vi "Init Objects by Type.vi"(8 "error in (no error)":errorcluster, 11 "Application Controller in":refnum<class "Application Controller.lvclass">) -> (0 "error out":errorcluster, 3 "Application Controller out":refnum<class "Application Controller.lvclass">)   [LabVIEW 2016, in "Application Controller.lvclass"]
uses:
  Application Controller.lvclass
  Sequence Elements/Sweep Sequence/Sweep.lvclass
  Sequence Elements/Record/Record.lvclass
  Application Controller.lvclass/Application Controller.ctl
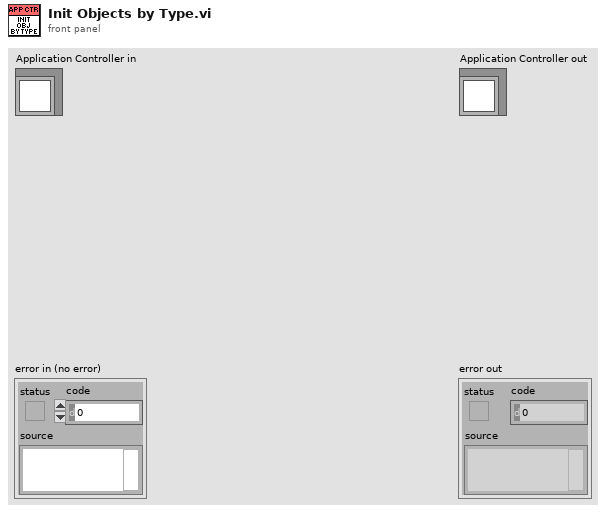
[diagram p1: front panel]
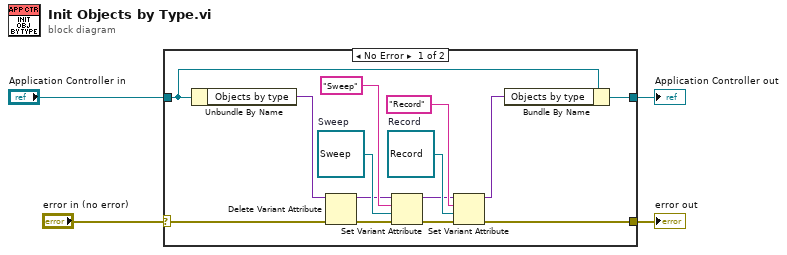
[diagram p0: block diagram]
diagram:
  n1 = case shown="No Error" "error in (no error)" {
    selector: "error in (no error)" -> [w6 w20]
    tunnel: [w5 w20] -> w3
    tunnel: [w8 w19] -> w1
    tunnel: "Application Controller in" -> [w18 w19]
    frame No Error {
      w12 = refnum<class "Record.lvclass"> refnum  # Record
      w16 = refnum<class "Sweep.lvclass"> refnum  # Sweep
      n2 = Unbundle By Name(w18) -> ("Objects by type"=w17:variant)
      n3 = Delete Variant Attribute(4:w6, 7:w17) -> (0:w14:errorcluster, 3:w13:variant)  [unwired: 1 in, 1 out]
      n4 = Set Variant Attribute(Variant=w13, name="Sweep", value=w16, error in=w14) -> (Variant out=w9:variant, error out=w10:errorcluster)  [unwired: 1 out]
      n5 = Set Variant Attribute(Variant=w9, name="Record", value=w12, error in=w10) -> (Variant out=w7:variant, error out=w5:errorcluster)  [unwired: 1 out]
      n6 = Bundle By Name(cluster=w18, "Objects by type"=w7) -> (w8:refnum<class "Application Controller.lvclass">)
    }
    frame Error {
    }
  }
  "error out" <- w3
  "Application Controller out" <- w1
